vi "Wheel Pivot.vi"(2 "y in":dbl, 3 "x in":dbl) -> (0 "y out":dbl, 1 "x out":dbl)   [LabVIEW 2013]
panel:
  in  "length/2":dbl=13.75
  in  "width/2":dbl=14.0
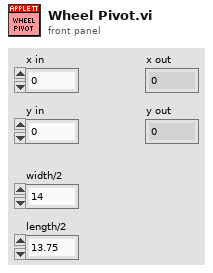
[diagram p1: front panel]
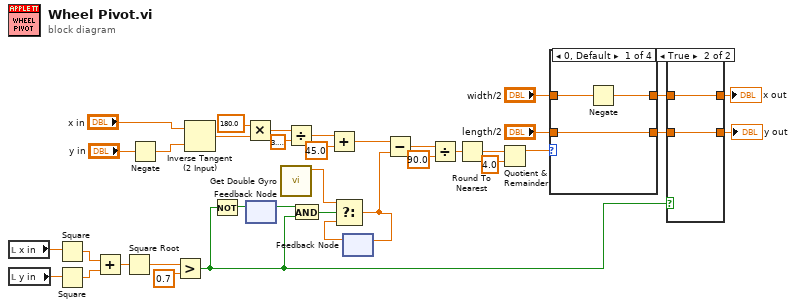
[diagram p0: block diagram]
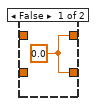
[diagram p2: hidden frame]
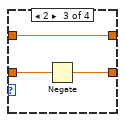
[diagram p4: hidden frame]
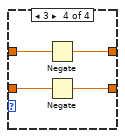
[diagram p5: hidden frame]
diagram:
  n1 = local read "x in"() -> (w19:dbl)
  n2 = local read "y in"() -> (w18:dbl)
  n3 = Square(x=w19) -> (x^2=w17:dbl)
  n4 = Square(x=w18) -> (x^2=w16:dbl)
  n5 = Add(x=w17, y=w16) -> (x+y=w15:dbl)
  n6 = Square Root(x=w15) -> (sqrt(x)=w14:dbl)
  n7 = Negate(x="y in") -> (-x=w29:dbl)
  n8 = Greater?(x=w14, y=0.7) -> (0:w6:bool)
  n9 = Inverse Tangent (2 Input)(1:w29, 2:"x in") -> (0:w28:dbl)
  n10 = Not(x=w6) -> (.not. x?=w8:bool)
  n11 = Multiply(x=180.0, y=w28) -> (x*y=w26:dbl)
  n12 = feedback-in #1(w8) -> ()
  n13 = feedback #1() -> (w7:bool)  [unwired: 1 in]
  n14 = call "Get Double Gyro.vi"() -> ("Angle"=w2:dbl)  [unwired: 10 in, 1 out]
  n15 = Divide(x=w26, y=3.141592653589793) -> (x/y=w22:dbl)
  n16 = And(x=w7, y=w6) -> (x .and. y?=w5:bool)
  n17 = Add(x=w22, y=45.0) -> (x+y=w20:dbl)
  n18 = feedback #2() -> (w4:dbl)  [unwired: 1 in]
  n19 = Select(t=w2, s=w5, f=w4) -> (s? t:f=w1:dbl)
  n20 = feedback-in #2(w1) -> ()
  n21 = Subtract(x=w20, y=w1) -> (x-y=w34:dbl)
  n22 = Divide(x=w34, y=90.0) -> (x/y=w32:dbl)
  n23 = Round To Nearest(number=w32) -> (nearest integer value=w31:dbl)
  n24 = Quotient & Remainder(x=w31, y=4.0) -> (x-y*floor(x/y)=w3:dbl)  [unwired: 1 out]
  n25 = case shown="0, Default" w3 {
    tunnel: "width/2" -> [w39 w41 w42 w48]
    tunnel: "length/2" -> [w37 w40 w44 w46]
    tunnel: [w38 w41 w42 w47] -> w13
    tunnel: [w37 w40 w43 w45] -> w11
    frame 0, Default {
      n26 = Negate(x=w39) -> (-x=w38:dbl)
    }
    frame 1 {
    }
    frame 2 {
      n27 = Negate(x=w44) -> (-x=w43:dbl)
    }
    frame 3 {
      n28 = Negate(x=w48) -> (-x=w47:dbl)
      n29 = Negate(x=w46) -> (-x=w45:dbl)
    }
  }
  n30 = case shown="True" w6 {
    tunnel: w13 -> [_ w51]
    tunnel: [w49 w51] -> w12
    tunnel: w11 -> [_ w50]
    tunnel: [w49 w50] -> w10
    frame False {
      w49 = 0.0 ("y")
    }
    frame True {
    }
  }
  "x out" <- w12
  "y out" <- w10
